vi "menuActivate.vi"(8 "error in (no error)":errorcluster, 10 "flatMenu[] in":T1, 11 "xceDataNode in":refnum<class "xceDataNode.lvclass">) -> (0 "error out":errorcluster, 2 "flatMenu[] out":T1, 3 "xceDataNode out":refnum<class "xceDataNode.lvclass">)   [LabVIEW 2013, in "xceDataNode.lvclass"]
doc: "Takes the relevent data of the xceDataNode, and produces an array which represents the menu options in the tree control."
uses:
  xceDataNode.lvclass
  _shared/flatMenu.ctl
  xceDataNode.lvclass/xceDataNode.ctl
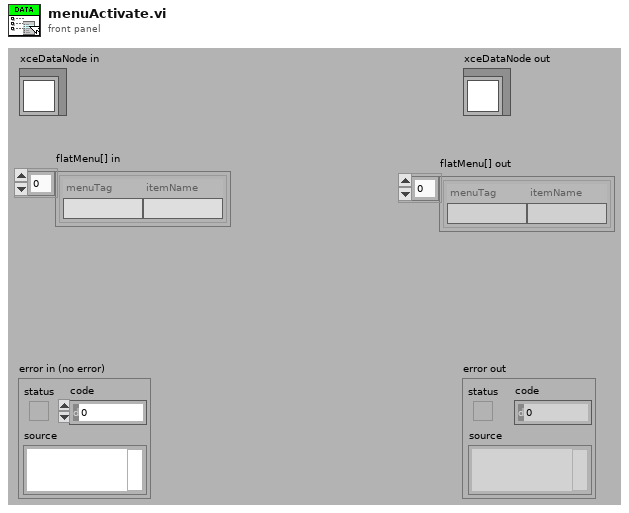
[diagram p1: front panel]
types:
  T1 = typedef "flatMenu.ctl" = cluster{"menuTag":string, "itemName":string}[]
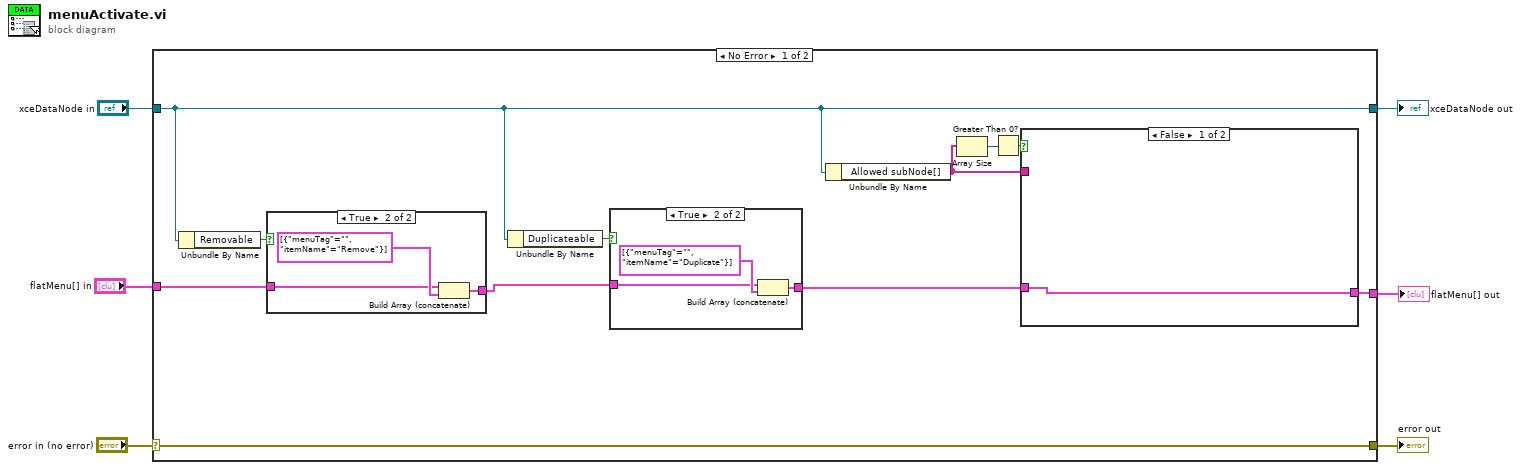
[diagram p0: block diagram]
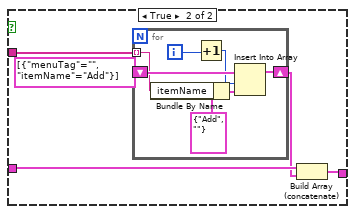
[diagram p2: hidden frame]
diagram:
  n1 = case shown="No Error" "error in (no error)" {
    selector: "error in (no error)" -> [w17 w39]
    tunnel: [w17 w39] -> w5
    tunnel: [w12 w38] -> w3
    tunnel: "xceDataNode in" -> [w12 w38]
    tunnel: "flatMenu[] in" -> [w15 _]
    tunnel: [w8 _] -> w1
    frame No Error {
      n2 = Unbundle By Name(w12) -> ("Removable"=w16:bool)
      n3 = case shown="True" w16 {
        tunnel: w15 -> [w34 w36]
        tunnel: [w34 w35] -> w13
        frame False {
        }
        frame True {
          n4 = Build Array (concatenate)(w36, T1 [{"menuTag"="", "itemName"="Remove"}] ("flatMenu[] in")) -> (w35:T1)
        }
      }
      n5 = Unbundle By Name(w12) -> ("Duplicateable"=w14:bool)
      n6 = case shown="True" w14 {
        tunnel: w13 -> [_ w32]
        tunnel: [_ w31] -> w7
        frame False {
        }
        frame True {
          n7 = Build Array (concatenate)(w32, T1 [{"menuTag"="", "itemName"="Duplicate"}] ("flatMenu[] in")) -> (w31:T1)
        }
      }
      n8 = Unbundle By Name(w12) -> ("Allowed subNode[]"=w9:string[])
      n9 = Array Size(array=w9) -> (size(s)=w10:i32)
      n10 = Greater Than 0?(x=w10) -> (x > 0?=w11:bool)
      n11 = case shown="False" w11 {
        tunnel: w9 -> [_ w22]
        tunnel: [w18 w19] -> w8
        tunnel: w7 -> [w18 w21]
        frame False {
        }
        frame True {
          n12 = for {
            shift-right: [w29] -> w20
            shift-left: T1 [{"menuTag"="", "itemName"="Add"}] ("flatMenu[] in") -> [w30]
            tunnel: w22 -> [w27] mode=indexing
            i -> [w25]
            n13 = Bundle By Name(cluster=cluster{"menuTag":string, "itemName":string} {"menuTag"="Add", "itemName"=""} ("new element/subarray"), "itemName"=w27) -> (w26:cluster{"menuTag":string, "itemName":string})
            n14 = Increment(x=w25) -> (x+1=w24:i32)
            n15 = Insert Into Array(array=w30, index=w24, new element=w26) -> (w29:T1)
          }
          n16 = Build Array (concatenate)(w21, w20) -> (w19:T1)
        }
      }
    }
    frame Error {
    }
  }
  "error out" <- w5
  "xceDataNode out" <- w3
  "flatMenu[] out" <- w1
